vi "Dryer Log GEA Data async.vi"(0 "Log File Type":T1, 1 "Header":string, 5 "Active Log File":string, 7 "Log File Folder":path, 11 "Error In":errorcluster) -> (15 "Error Out":errorcluster)   [LabVIEW 2014]
uses:
  Common/LabVIEW GEA2 Toolkit/LabVIEW_GEA2_Toolkit.lvlibp
  Common/LabVIEW GEA2 Toolkit/LabVIEW_GEA2_Toolkit.lvlibp/type defs/Data In.ctl
  type defs/Dryer_Log_State.ctl
  type defs/Log_File_Type.ctl
panel:
  in  "Board Index":i32
  out "Board ID":string
  out "Init Debug File":bool
  out "Log":string
  in  "Input Data":T2={"Source"=228, "Destination"=0, "Command"=0, "Message"=""} {"Command" format="%02x"; "Destination" format="%02x"; "Source" format="%02x"}
  in  "Stop":bool
  in  "Send":bool
  # "Dryer Data Logger"
  # "To see error data, scroll down."
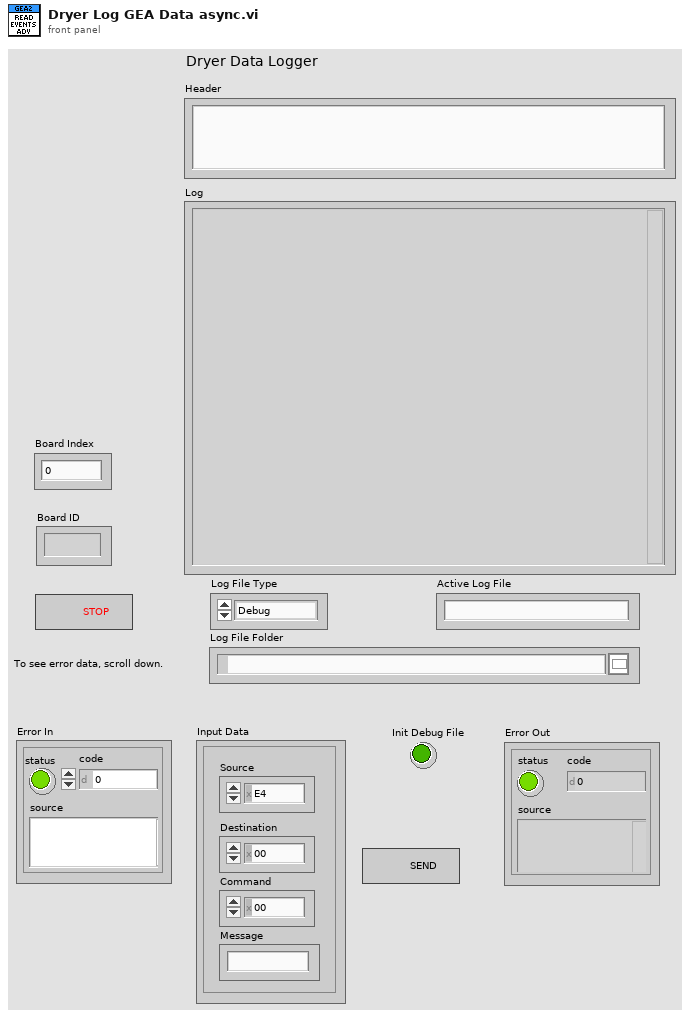
[diagram p1: front panel]
types:
  T1 = typedef "Log_File_Type.ctl" = enum16{"Debug", "Bus Traffic"}
  T2 = typedef "LabVIEW_GEA2_Toolkit.lvlibp/Data In.ctl" = cluster{"Source":u8, "Destination":u8, "Command":u8, "Message":string}
  T3 = typedef "Dryer_Log_State.ctl" = enum16{"Close", "Log", "Open"}
  T4 = enum16{"open", "replace", "create", "open or create", "replace or create", "replace or create with confirmation"}
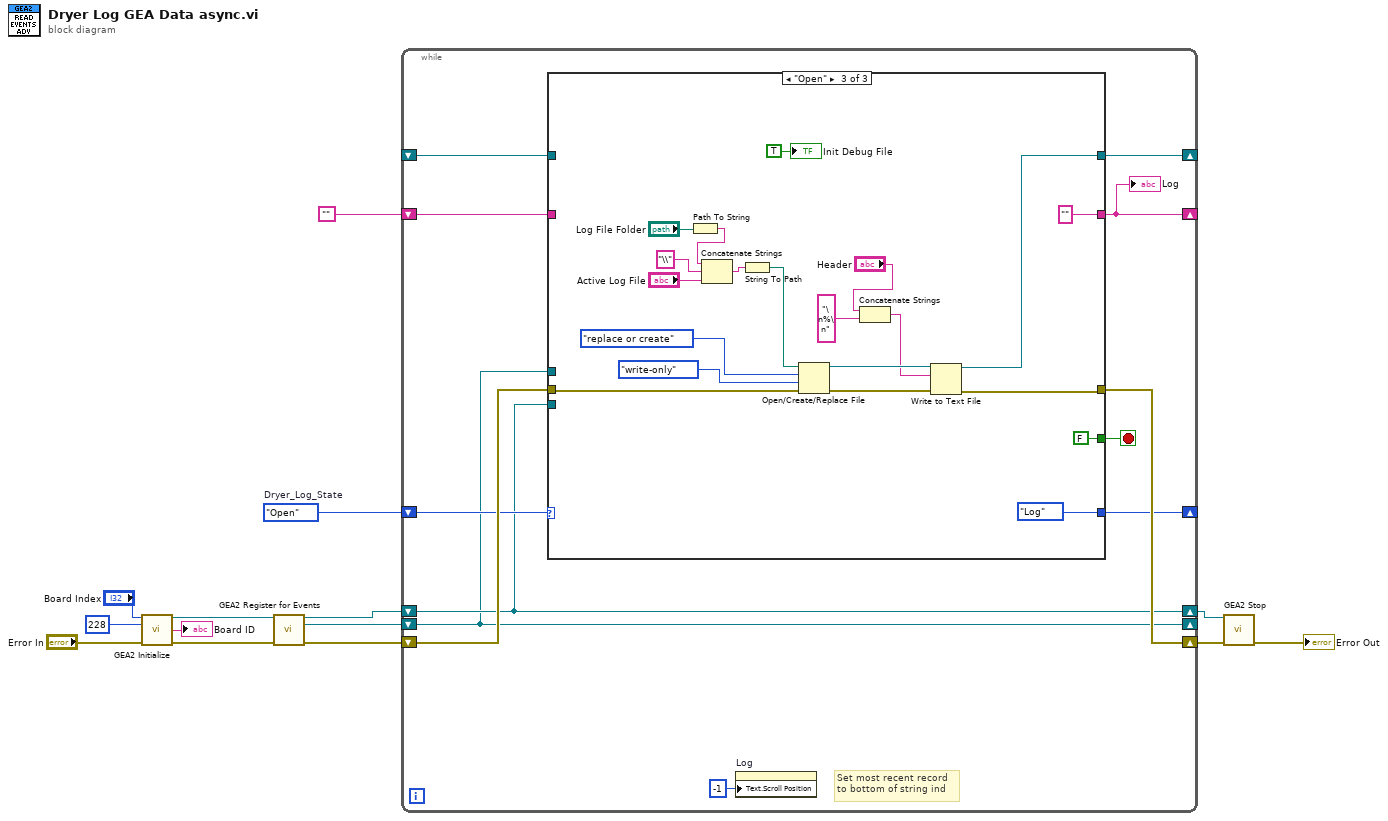
[diagram p0: block diagram]
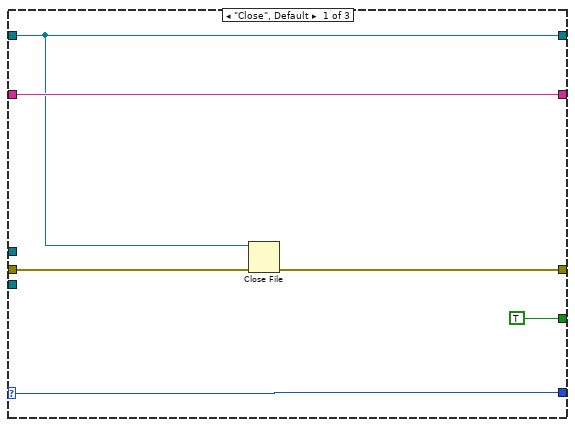
[diagram p2: hidden frame]
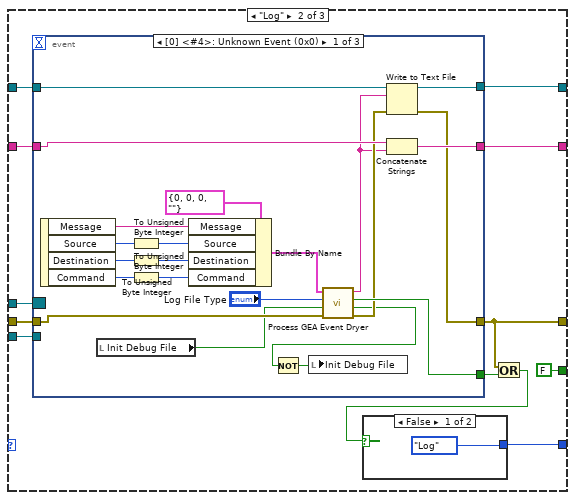
[diagram p3: hidden frame]
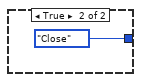
[diagram p4: hidden frame]
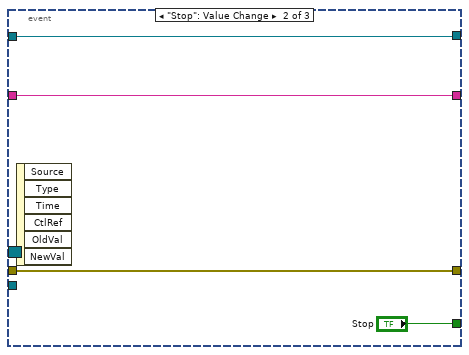
[diagram p5: hidden frame]
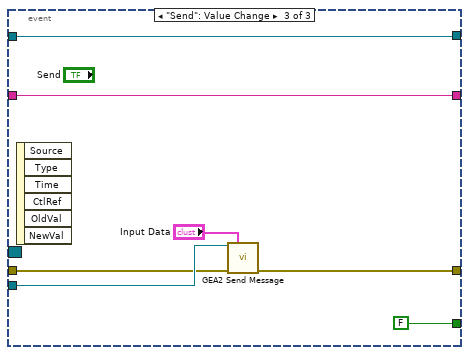
[diagram p6: hidden frame]
diagram:
  w4 = Dryer_Log_State."Open"  # Dryer_Log_State
  n1 = call "GEA2 Initialize.vi"("Board Index"="Board Index", "Source Address"=u8 228, "error in"="Error In") -> ("GEA2 Reference Out"=w12:refnum<k24>, "Board ID"=→"Board ID":string, "error out"=w13:errorcluster)  [unwired: 10 in]
  n2 = call "GEA2 Register for Events.vi"("GEA2 Reference In"=w12, "Error In"=w13) -> ("GEA2 Reference Out"=w9:refnum<k24>, "Event Registration Refnum"=w7:refnum<event-registration>, "Error Out"=w8:errorcluster)  [unwired: 11 in]
  n3 = while {
    shift-right: [w24] -> w11
    shift-left: w8 -> [w25]
    shift-right: [w22] -> _
    shift-left: "" -> [w23]
    shift-right: [w19] -> _
    shift-left: _ -> [w18]
    shift-right: [w17] -> _
    shift-left: w4 -> [w20]
    shift-right: [w16] -> w3
    shift-left: w9 -> [w16]
    shift-right: [w15] -> _
    shift-left: w7 -> [w15]
    stop <- w26 stop-if-true
    # "Set most recent record\nto bottom of string ind"
    n4 = case shown="\"Open\"" w20 {
      selector: w20 -> [w27 _ _]
      tunnel: [TRUE FALSE FALSE] -> w26
      tunnel: w15 -> [_ w44 _]
      tunnel: w25 -> [w31 w43 w98]
      tunnel: w16 -> [_ w42 _]
      tunnel: [w30 w34 w86] -> w24
      tunnel: w23 -> [w32 w41 _]
      tunnel: [w32 w40 ""] -> w22
      tunnel: [w29 w37 w84] -> w19
      tunnel: w18 -> [w29 w38 _]
      tunnel: [w27 w33 Dryer_Log_State."Log" ("Dryer_Log_State")] -> w17
      frame "Close", Default {
        n5 = Close File(refnum=w29, error in=w31) -> (error out=w30:errorcluster)  [unwired: 1 out]
      }
      frame "Log" {
        n6 = event shown="[0] <#4>: Unknown Event (0x0)" {
          selector: w44 -> [_ _ _]
          dyn-events: _ -> [_ _ _]
          timeout: _ -> [_ _ _]
          tunnel: w43 -> [w59 w71 w78]
          tunnel: [w53 w71 w77] -> w34
          tunnel: w42 -> [_ _ w79]
          tunnel: w41 -> [w56 w70 w75]
          tunnel: [w58 w70 w75] -> w40
          tunnel: [w57 "Stop" FALSE ("Stop")] -> w39
          tunnel: w38 -> [w55 w69 w73]
          tunnel: [w52 w69 w73] -> w37
          event User Event {
            n7 = event-data() -> ("Message"=w62:string, "Source"=w63:u8, "Destination"=w64:u8, "Command"=w65:u8)  [unwired: 1 in]
            n8 = local read "Init Debug File"() -> (w49:bool)
            n9 = To Unsigned Byte Integer(number=w63) -> (unsigned 8bit integer=w67:u8)
            n10 = To Unsigned Byte Integer(number=w64) -> (unsigned 8bit integer=w68:u8)
            n11 = To Unsigned Byte Integer(number=w65) -> (unsigned 8bit integer=w66:u8)
            n12 = Bundle By Name(cluster=T2 {"Source"=0, "Destination"=0, "Command"=0, "Message"=""} ("GEA2 Data In"), "Message"=w62, "Source"=w67, "Destination"=w68, "Command"=w66) -> (w60:T2)
            n13 = call "Process GEA Event Dryer.vi"("error in (no error)"=w59, "Init Debug File"=w49, "Log File Type"="Log File Type", "GEA2 Data In"=w60) -> ("error out"=w54:errorcluster, "Debug File Initialized"=w47:bool, "End Cycle"=w57:bool, "Output String"=w51:string)  [unwired: 4 in]
            n14 = Not(x=w47) -> (.not. x?=w48:bool)
            n15 = local write "Init Debug File"(w48) -> ()
            n16 = Write to Text File(file (use dialog)=w55, text=w51, error in=w54) -> (refnum out=w52:refnum<file>, error out=w53:errorcluster)  [unwired: 1 in, 1 out]
            n17 = Concatenate Strings(w56, w51) -> (w58:string)
          }
          event "Stop": Value Change {
            n18 = event-data() -> ()  [unwired: 1 in, 6 out]
          }
          event "Send": Value Change {
            n19 = event-data() -> ()  [unwired: 1 in, 6 out]
            n20 = call "GEA2 Send Message.vi"("GEA2 Reference In"=w79, "Input Data"="Input Data", "Error In"=w78) -> ("Error Out"=w77:errorcluster)  [unwired: 11 in, 1 out]
          }
        }
        n21 = Or(x=w34, y=w39) -> (x .or. y?=w36:bool)
        n22 = case shown="False" w36 {
          tunnel: [Dryer_Log_State."Log" ("Dryer_Log_State") Dryer_Log_State."Close" ("Dryer_Log_State")] -> w33
          frame False {
          }
          frame True {
          }
        }
      }
      frame "Open" {
        n23 = Path To String(path="Log File Folder") -> (string=w93:string)
        n24 = Concatenate Strings(w93, "\\" ("string"), "Active Log File") -> (w91:string)
        n25 = String To Path(string=w91) -> (path=w90:path)
        n26 = Open/Create/Replace File(file path (use dialog)=w90, error in=w98, operation (0:open)=T4."replace or create", access (0:read/write)=enum16{"read/write", "read-only", "write-only"}."write-only") -> (refnum out=w85:refnum<file>, error out=w87:errorcluster)  [unwired: 2 in, 1 out]
        n27 = Concatenate Strings("Header", "\n%\n" ("string")) -> (w82:string)
        n28 = Write to Text File(file (use dialog)=w85, text=w82, error in=w87) -> (refnum out=w84:refnum<file>, error out=w86:errorcluster)  [unwired: 1 in, 1 out]
        "Init Debug File" <- TRUE ("Init Log File")
      }
    }
    "Log" <- w22
    n29 = property on="Log" class="Str"("Text.Scroll Position"=-1) -> ()  [unwired: 2 in, 2 out]
  }
  n30 = call "GEA2 Stop.vi"("GEA2 Reference In"=w3, "Error In"=w11) -> ("Error Out"=→"Error Out":errorcluster)  [unwired: 13 in]
